vi "CreateLVContextMenu.vi"() -> ()   [LabVIEW 2016]
uses:
  TypeDefs/LV Version Details.ctl
panel:
  out "LV Version Details":T1[](array[typedef])
  in  "Create":bool
  # "The application adds a windows right click context menu for all the versions of LabVIEW\ninstalled on this PC. This makes it handy when you want to open a LabVIEW file in a particular\nversion of LabVIEW instead of the traditional method of File ->Open.\n\nInstructions\n\n1. When you run this application, it lists all the LabVIEW versions installed on this PC.\n2. Clicking on \"Create Context Menus\" button, adds a right click context menu for all the versions.\n3. If you see any erros, check if you are an admin account on this PC or run as admin."
  # "Sample"
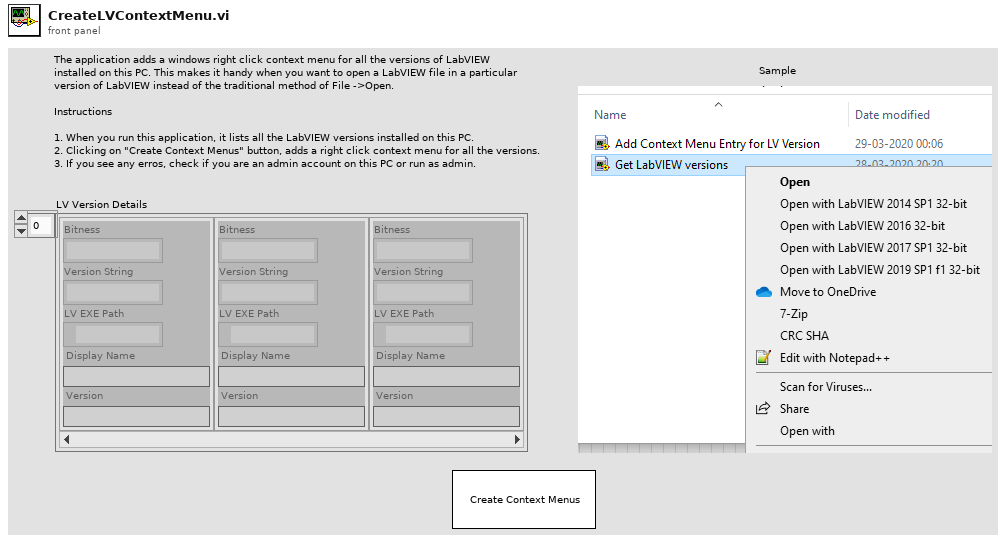
[diagram p1: front panel]
types:
  T1 = typedef "LV Version Details.ctl" = cluster{"Bitness":string, "Version String":string, "LV EXE Path":path, "Display Name":string, "Version":string}
  T2 = enum32{"Invalid", "Standard", "Closed", "Hidden", "Minimized", "Maximized"}
  T3 = enum32{"invalid app kind", "Development System", "Run Time System", "Student Edition", "Embedded LabVIEW", "Evaluation", "Custom"}
  T4 = cluster{"Core":cluster{"Current VI Reference":refnum<vi>, "Close Panel on Exit?":bool}, "Your Boolean data":bool, "Your string data":string, "LV Version Details":T1[]}
  T5 = cluster{"Current VI Reference":refnum<vi>, "Close Panel on Exit?":bool}
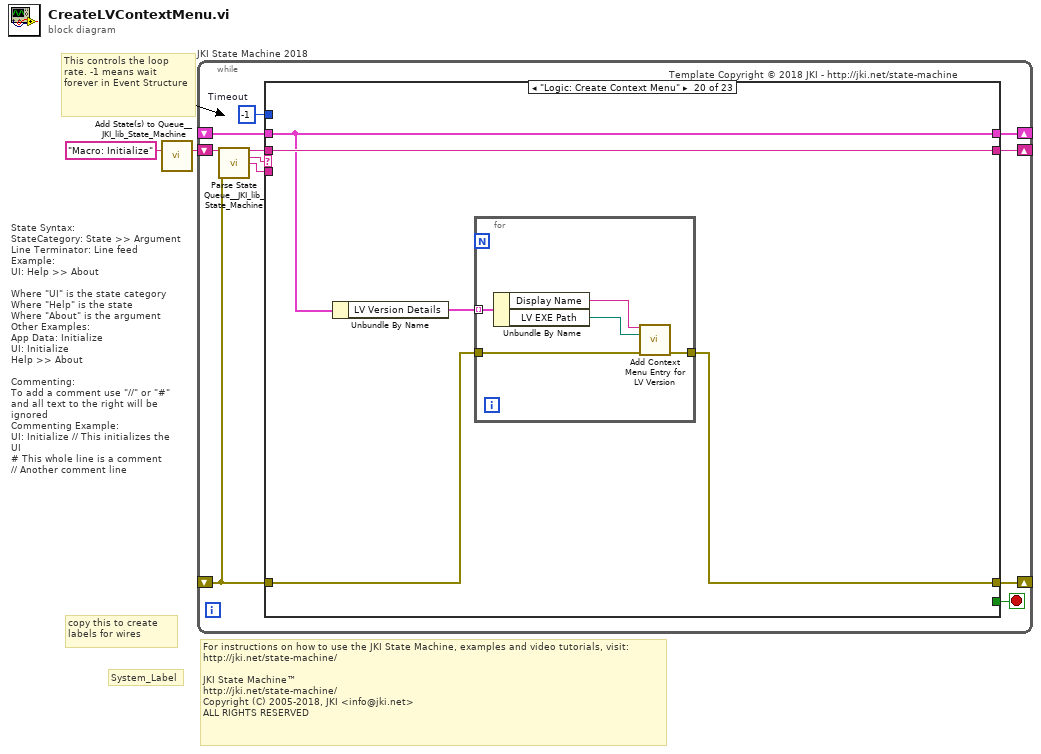
[diagram p0: block diagram]
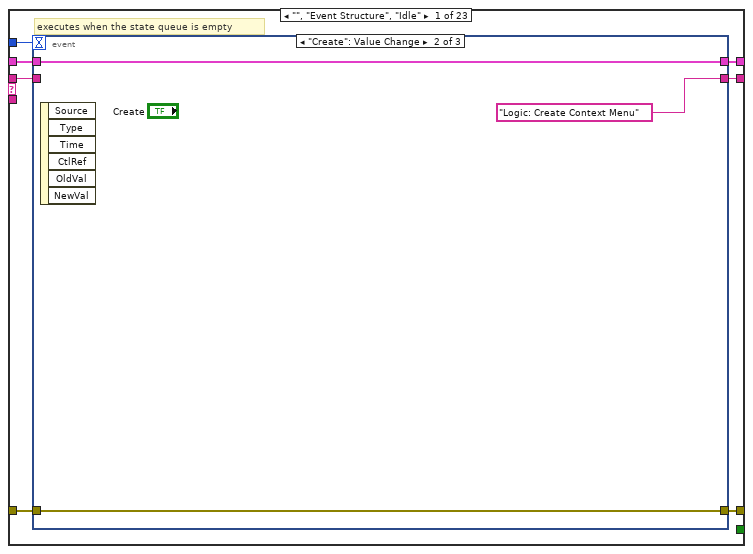
[diagram p2: hidden frame]
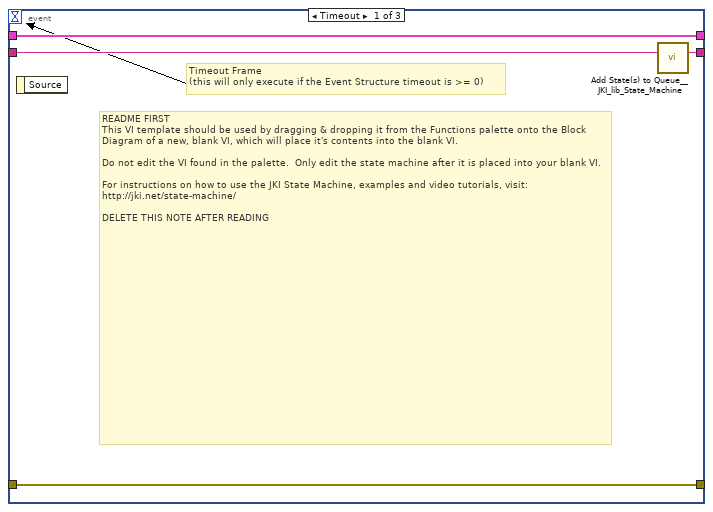
[diagram p3: hidden frame]
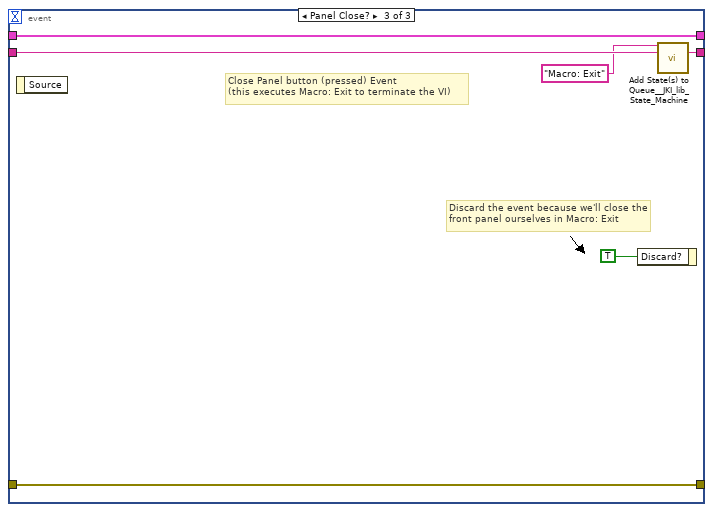
[diagram p4: hidden frame]
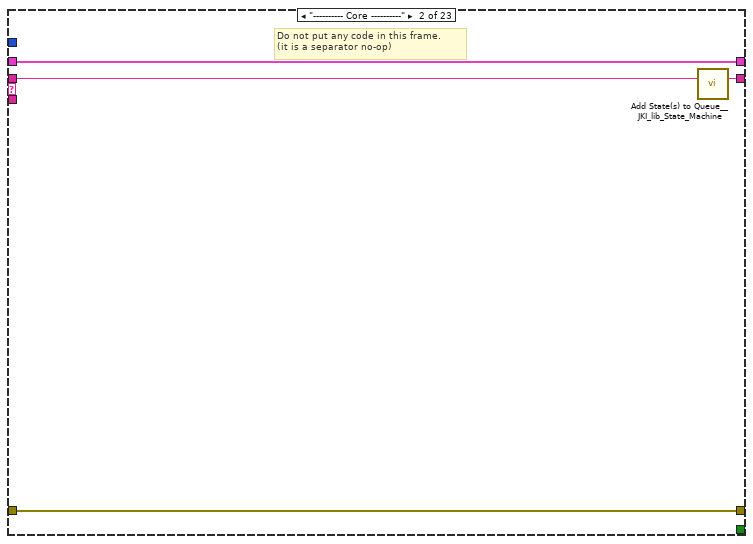
[diagram p5: hidden frame]
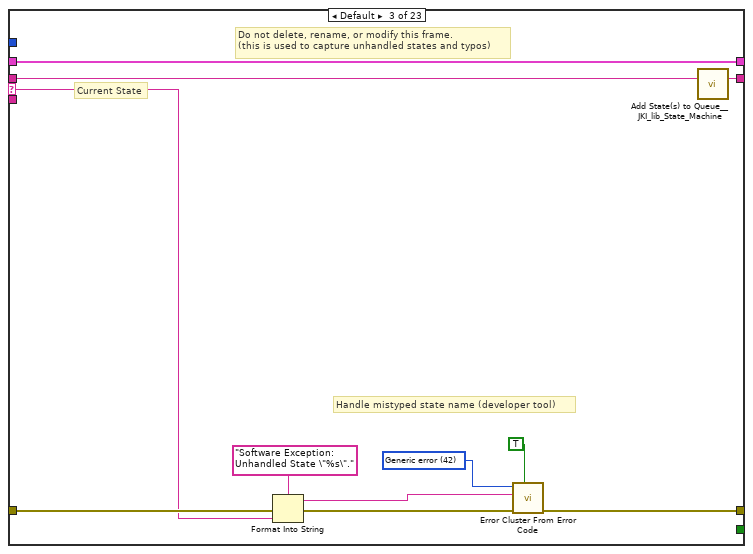
[diagram p6: hidden frame]
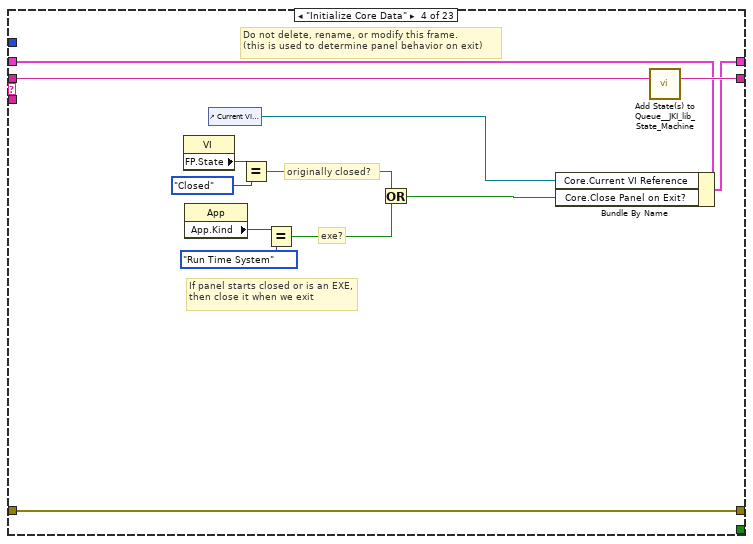
[diagram p7: hidden frame]
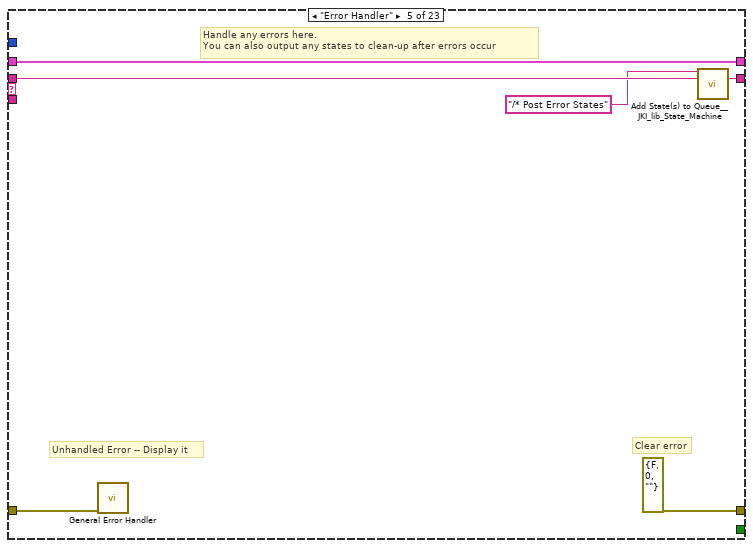
[diagram p8: hidden frame]
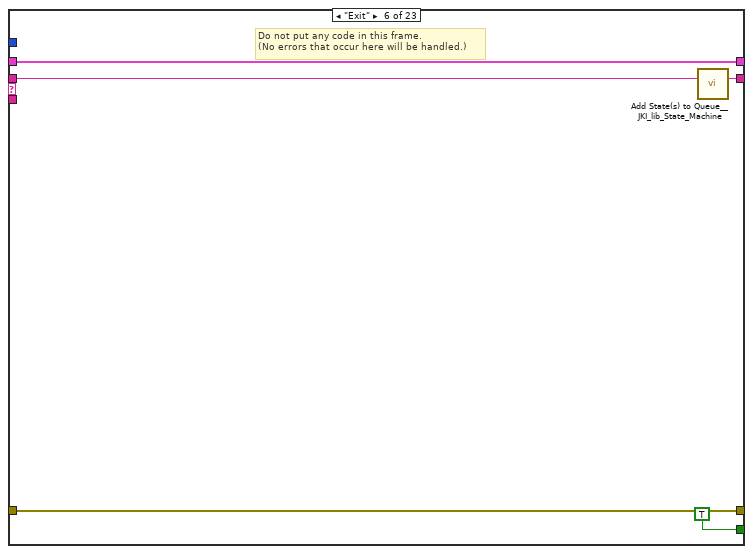
[diagram p9: hidden frame]
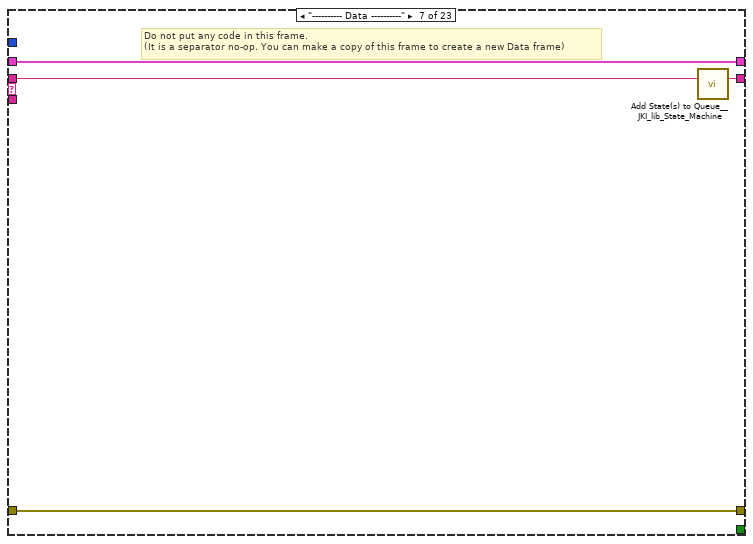
[diagram p10: hidden frame]
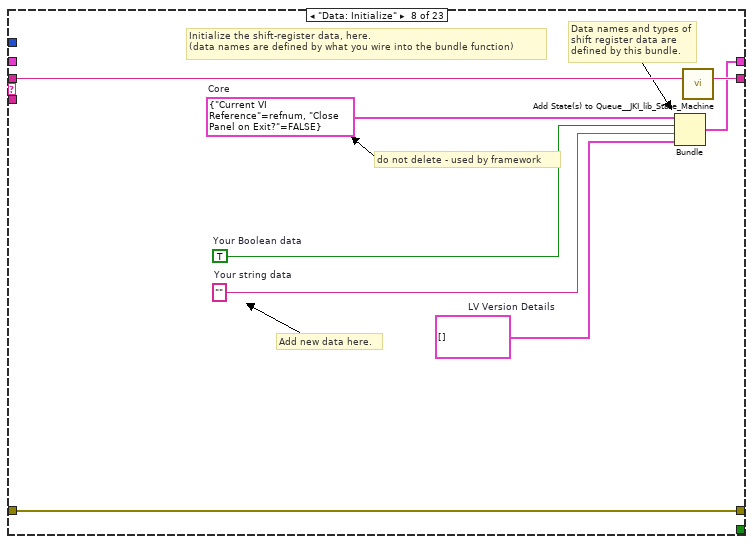
[diagram p11: hidden frame]
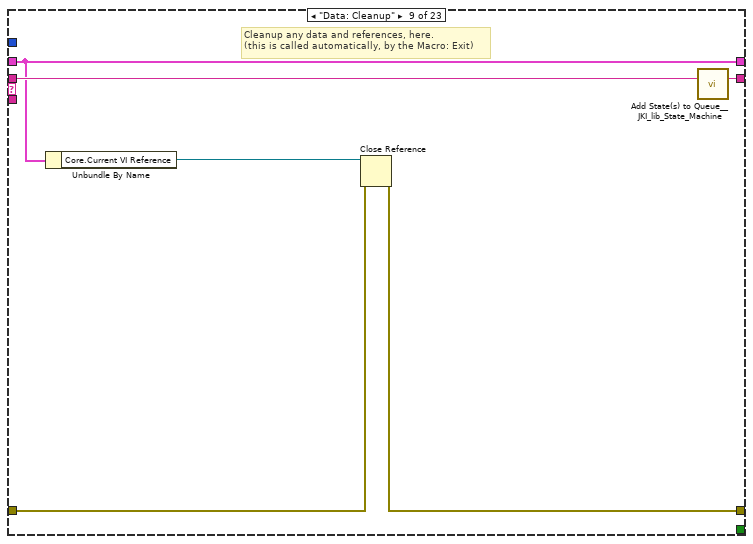
[diagram p12: hidden frame]
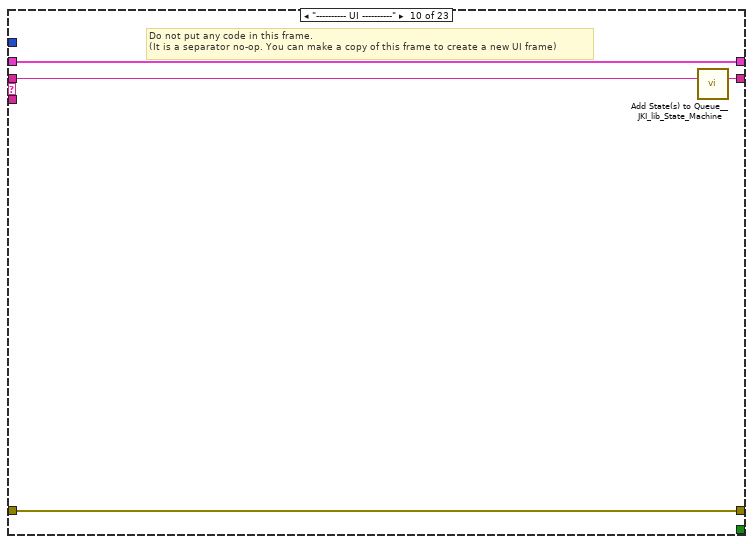
[diagram p13: hidden frame]
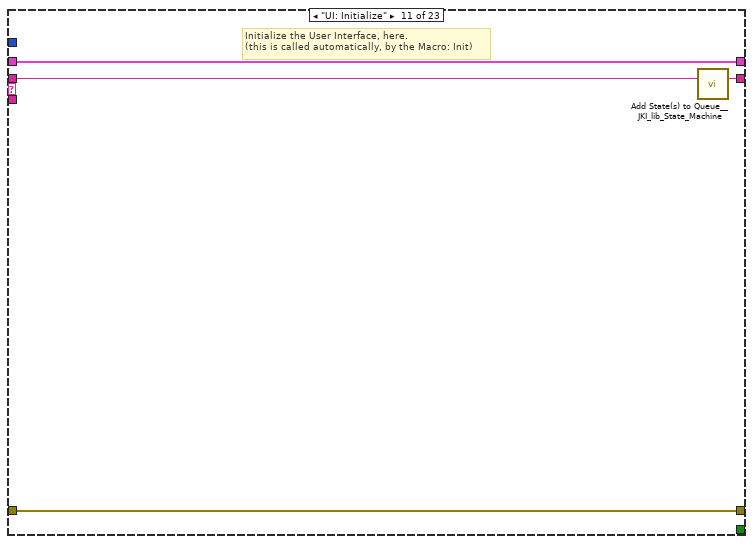
[diagram p14: hidden frame]
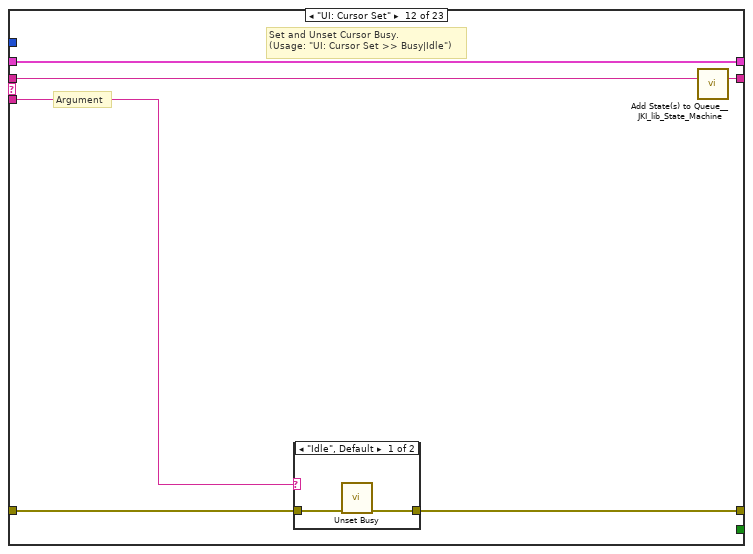
[diagram p15: hidden frame]
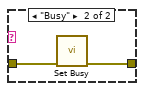
[diagram p16: hidden frame]
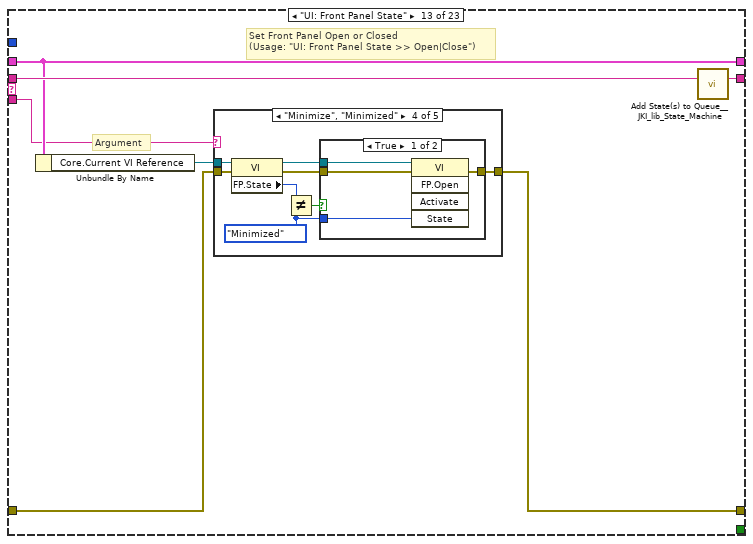
[diagram p17: hidden frame]
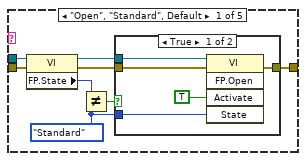
[diagram p18: hidden frame]
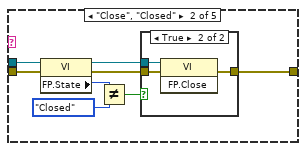
[diagram p20: hidden frame]
diagram:
  # "For instructions on how to use the JKI State Machine, examples and video tutorials, visit:\nhttp://jki.net/state-machine/\n\nJKI State Machine™\nhttp://jki.net/state-machine/\nCopyright (C) 2005-2018, JKI <info@jki.net>\nALL RIGHTS RESERVED"
  # "State Syntax:\nStateCategory: State >> Argument\nLine Terminator: Line feed\nExample:\nUI: Help >> About\n\nWhere \"UI\" is the state category\nWhere \"Help\" is the state\nWhere \"About\" is the argument\nOther Examples:\nApp Data: Initialize\nUI: Initialize\nHelp >> About\n\nCommenting:\nTo add a comment use \"//\" or \"#\" and all text to the right will be ignored\nCommenting Example:\nUI: Initialize // This initializes the UI\n# This whole line is a comment\n// Another comment line"
  # "copy this to create labels for wires"
  # "This controls the loop rate. -1 means wait forever in Event Structure"
  # "System_Label"
  n1 = call <vilib>:"Add State(s) to Queue__JKI_lib_State_Machine.vi"("State(s) in (\"\")"="Macro: Initialize") -> ("States Out"=w2:string)  [unwired: 14 in]
  n2 = while "JKI State Machine 2018" {
    shift-right: [w6] -> _
    shift-left: _ -> [w5]
    shift-right: [w9] -> _
    shift-left: _ -> [w3]
    shift-right: [w8] -> _
    shift-left: w2 -> [w10]
    stop <- w7 stop-if-true
    w4 = -1  # Timeout
    # "Template Copyright © 2018 JKI - http://jki.net/state-machine"
    n3 = call <vilib>:"Parse State Queue__JKI_lib_State_Machine.vi"("State Queue"=w10, "Error In (no error)"=w3) -> ("Remaining States"=w12:string, "Current State"=w13:string, "Arguments"=w11:string)  [unwired: 11 in]
    n4 = case shown="\"Logic: Create Context Menu\"" w13 {
      selector: w13 -> [_ _ w38 _ _ _ _ _ _ _ _ _ _ _ _ _ _ _ _ _ _ _ _]
      tunnel: w12 -> [w20 w37 w42 w61 w67 w72 w76 w84 w90 w94 w98 w104 w115 w183 w188 w193 w203 w205 _ w217 w226 w230 w234]
      tunnel: w11 -> [_ _ _ _ _ _ _ _ _ _ _ w99 w109 _ _ _ _ _ _ _ _ _ _]
      tunnel: w5 -> [w18 w34 w40 w54 w64 w70 w73 _ w85 w91 w96 w102 w111 w182 w185 w190 w200 w206 w209 w216 w223 w227 w231]
      tunnel: [w17 w35 w44 w58 errorcluster {"status"=FALSE, "code"=0, "source"=""} ("error out") w69 w74 w81 w86 w92 w95 w100 w112 w184 w186 w191 w201 w204 w211 w213 w224 w228 w232] -> w9
      tunnel: w3 -> [w16 w35 w43 w58 w63 w69 w74 w81 w87 w92 w95 w101 w113 w184 w186 w191 w201 w204 w212 w215 w224 w228 w232]
      tunnel: [w19 w36 w41 w60 w66 w71 w75 w83 w89 w93 w97 w103 w114 w183 w187 w192 w202 w205 "UI: Display All LabVIEW Versions" w217 w225 w229 w233] -> w8
      tunnel: [_ _ _ _ _ TRUE _ _ _ _ _ _ _ _ _ _ _ _ _ _ _ _ _] -> w7
      tunnel: [w15 w34 w40 w59 w64 w70 w73 w82 w85 w91 w96 w102 w111 w182 w185 w190 w200 w206 w208 w216 w223 w227 w231] -> w6
      tunnel: w4 -> [w14 _ _ _ _ _ _ _ _ _ _ _ _ _ _ _ _ _ _ _ _ _ _]
      frame "", "Event Structure", "Idle" {
        # "executes when the state queue is empty"
        n5 = event shown="[1] \"Create\": Value Change" {
          selector: _ -> [_ _ _]
          dyn-events: _ -> [_ _ _]
          timeout: w14 -> [_ _ _]
          tunnel: w20 -> [w24 _ w33]
          tunnel: [w23 "Logic: Create Context Menu" ("States Out") w32] -> w19
          tunnel: w18 -> [w21 w26 w30]
          tunnel: [w22 w27 w31] -> w17
          tunnel: w16 -> [w22 w27 w31]
          tunnel: [w21 w26 w30] -> w15
          event Timeout {
            # "README FIRST\nThis VI template should be used by dragging & dropping it from the Functions palette onto the Block Diagram of a new, blank VI, which will place it's contents into the blank VI.\n\nDo not edit the VI found in the palette.  Only edit the state machine after it is placed into your blank VI.\n\nFor instructions on how to use the JKI State Machine, examples and video tutorials, visit:\nhttp://jki.net/state-machine/\n\nDELETE THIS NOTE AFTER READING"
            # "Timeout Frame\n(this will only execute if the Event Structure timeout is >= 0)"
            n6 = event-data() -> ()  [unwired: 1 in, 1 out]
            n7 = call <vilib>:"Add State(s) to Queue__JKI_lib_State_Machine.vi"("State(s) in (\"\")"=w24) -> ("States Out"=w23:string)  [unwired: 14 in]
          }
          event "Create": Value Change {
            n8 = event-data() -> ()  [unwired: 1 in, 6 out]
          }
          event Panel Close? {
            # "Discard the event because we'll close the front panel ourselves in Macro: Exit"
            # "Close Panel button (pressed) Event\n(this executes Macro: Exit to terminate the VI)"
            n9 = event-data() -> ()  [unwired: 1 in, 1 out]
            n10 = event-data("Discard?"=TRUE) -> ()  [unwired: 1 in, 1 out]
            n11 = call <vilib>:"Add State(s) to Queue__JKI_lib_State_Machine.vi"("State(s) in Front (\"\")"="Macro: Exit", "State(s) in (\"\")"=w33) -> ("States Out"=w32:string)  [unwired: 13 in]
          }
        }
      }
      frame "---------- Core ----------" {
        # "Do not put any code in this frame.\n(it is a separator no-op)"
        n12 = call <vilib>:"Add State(s) to Queue__JKI_lib_State_Machine.vi"("State(s) in (\"\")"=w37) -> ("States Out"=w36:string)  [unwired: 14 in]
      }
      frame Default {
        w47 = 42 items=["No error", "Argument error", "Memory is full", "Out of zone", "End of file", "File already open", "Generic file I/O error", "File not found", "File permission error", "Disk is full", "Duplicate path", "Too many files open", "System feature not enabled", "Resource file not found", "Cannot add resource", "Resource not found", "Image not found", "Image memory error", "Pen does not exist", "Config type invalid", "Config token not found", "Config parse error", "Config memory error", "Bad external code format", "Bad external code offset", "External code not present", "Null window", "Destroy window error", "Null menu", "Print aborted", "Bad print record", "Print driver error", "Windows error during printing", "Memory error during printing", "Print dialog error", "Generic print error", "Invalid device refnum", "Device not found", "Device parameter error", "Device unit error", "Cannot open device", "Device call aborted", "Generic error", "Cancelled by user", "Object ID too low", "Object ID too high", "Object not in heap", "Unknown heap", "Unknown object (invalid DefProc)", "Unknown object (DefProc not in table)", "Message out of range", "Invalid (null) method", "Unknown message", "Manager call not supported", "Bad address", "Network operation in progress", "Network operation timed out", "Connection is busy", "Network attribute not supported", "Network error", "Address in use", "System out of memory", "Connection aborted", "Connection refused", "Not connected", "Already connected", "Connection closed", "Initialization error (interapplication manager)", "Bad occurrence", "Wait on unbound occurrence handler", "Occurrence queue overflow", "Datalog type conflict", "Unused", "Unrecognized type (interapplication manager)", "Memory corrupt", "Failed to make temporary DLL", "Old CIN version", "Drag socket not found", "Failed to load drop-object", "Failed to register OLE object", "Failed to release OLE object", "Format specifier type mismatch", "Unknown format specifier", "Too few format specifiers", "Too many format specifiers", "Scan failed", "Newer CIN version", "Error converting to variant", "Runtime menu error", "Password tampered", "Variant attribute not found", "Incompatible variant data type", "Event data is not available", "Event Store is not present", "Occurrence is not found", "Event Queue is not created", "Event info is not available", "Refnum passed is NULL", "Error retrieving Class GUID", "Error retrieving CoClass GUID", "Error retrieving TypeLib GUID.", "Bad built application magic bytes.", "Specific driver is different from the specific driver associated with the Logical Name.", "There is no session opened to the class driver.", "Max Error", "MAX - Error with config objects", "MAX - Error loading configuration", "MAX - Group not supported"]
        # "Current State"
        # "Do not delete, rename, or modify this frame.\n(this is used to capture unhandled states and typos)"
        # "Handle mistyped state name (developer tool)"
        n13 = Format Into String(format string="Software Exception: Unhandled State \"%s\"." ("message"), error in=w43, w38) -> (resulting string=w46:string, error out=w45:errorcluster)  [unwired: 1 in]
        n14 = call <vilib>:"Error Cluster From Error Code.vi"("show call chain? (False)"=TRUE, "error in (no error)"=w45, "error message (\"\")"=w46, "error code (0)"=w47) -> ("error out"=w44:errorcluster)  [unwired: 5 in]
        n15 = call <vilib>:"Add State(s) to Queue__JKI_lib_State_Machine.vi"("State(s) in (\"\")"=w42) -> ("States Out"=w41:string)  [unwired: 14 in]
      }
      frame "Initialize Core Data" {
        # "Do not delete, rename, or modify this frame.\n(this is used to determine panel behavior on exit)"
        # "originally closed?"
        # "exe?"
        # "If panel starts closed or is an EXE, then close it when we exit"
        n16 = property class="VI"() -> ("FP.State"=w51:T2)  [unwired: 2 in, 2 out]
        n17 = property class="App"() -> ("App.Kind"=w57:T3)  [unwired: 2 in, 2 out]
        n18 = control-ref of="Current VI Reference"() -> (w52:refnum<vi>)
        n19 = Equal?(x=w51, y=T2."Closed" ("Front Panel Window:State")) -> (x = y?=w49:bool)
        n20 = Equal?(x=w57, y=T3."Run Time System" ("Application:Kind")) -> (x = y?=w55:bool)
        n21 = Or(x=w49, y=w55) -> (x .or. y?=w53:bool)
        n22 = Bundle By Name(cluster=w54, "Core.Current VI Reference"=w52, "Core.Close Panel on Exit?"=w53) -> (w59:T4)
        n23 = call <vilib>:"Add State(s) to Queue__JKI_lib_State_Machine.vi"("State(s) in (\"\")"=w61) -> ("States Out"=w60:string)  [unwired: 14 in]
      }
      frame "Error Handler" {
        # "Unhandled Error -- Display it"
        # "Handle any errors here.\nYou can also output any states to clean-up after errors occur"
        # "Clear error"
        n24 = call <vilib>:"General Error Handler.vi"("error in (no error)"=w63) -> ()  [unwired: 10 in, 5 out]
        n25 = call <vilib>:"Add State(s) to Queue__JKI_lib_State_Machine.vi"("State(s) in Front (\"\")"="/* Post Error States", "State(s) in (\"\")"=w67) -> ("States Out"=w66:string)  [unwired: 13 in]
      }
      frame "Exit" {
        # "Do not put any code in this frame.\n(No errors that occur here will be handled.)"
        n26 = call <vilib>:"Add State(s) to Queue__JKI_lib_State_Machine.vi"("State(s) in (\"\")"=w72) -> ("States Out"=w71:string)  [unwired: 14 in]
      }
      frame "---------- Data ----------" {
        # "Do not put any code in this frame.\n(It is a separator no-op. You can make a copy of this frame to create a new Data frame)"
        n27 = call <vilib>:"Add State(s) to Queue__JKI_lib_State_Machine.vi"("State(s) in (\"\")"=w76) -> ("States Out"=w75:string)  [unwired: 14 in]
      }
      frame "Data: Initialize" {
        w77 = T1[] []  # LV Version Details
        w78 = T5 {"Current VI Reference"=refnum, "Close Panel on Exit?"=FALSE}  # Core
        w80 = TRUE  # Your Boolean data
        w79 = ""  # Your string data
        # "do not delete - used by framework"
        # "Add new data here."
        # "Data names and types of shift register data are defined by this bundle."
        # "Initialize the shift-register data, here.\n(data names are defined by what you wire into the bundle function)"
        n28 = Bundle("Core"=w78, "Your Boolean data"=w80, "Your string data"=w79, "LV Version Details"=w77) -> (w82:T4)  [unwired: 1 in]
        n29 = call <vilib>:"Add State(s) to Queue__JKI_lib_State_Machine.vi"("State(s) in (\"\")"=w84) -> ("States Out"=w83:string)  [unwired: 14 in]
      }
      frame "Data: Cleanup" {
        # "Cleanup any data and references, here.\n(this is called automatically, by the Macro: Exit)"
        n30 = Unbundle By Name(w85) -> ("Core.Current VI Reference"=w88:refnum<vi>)
        n31 = Close Reference(reference=w88, error in (no error)=w87) -> (error out=w86:errorcluster)
        n32 = call <vilib>:"Add State(s) to Queue__JKI_lib_State_Machine.vi"("State(s) in (\"\")"=w90) -> ("States Out"=w89:string)  [unwired: 14 in]
      }
      frame "---------- UI ----------" {
        # "Do not put any code in this frame.\n(It is a separator no-op. You can make a copy of this frame to create a new UI frame)"
        n33 = call <vilib>:"Add State(s) to Queue__JKI_lib_State_Machine.vi"("State(s) in (\"\")"=w94) -> ("States Out"=w93:string)  [unwired: 14 in]
      }
      frame "UI: Initialize" {
        # "Initialize the User Interface, here.\n(this is called automatically, by the Macro: Init)"
        n34 = call <vilib>:"Add State(s) to Queue__JKI_lib_State_Machine.vi"("State(s) in (\"\")"=w98) -> ("States Out"=w97:string)  [unwired: 14 in]
      }
      frame "UI: Cursor Set" {
        # "Argument"
        # "Set and Unset Cursor Busy.\n(Usage: \"UI: Cursor Set >> Busy|Idle\")"
        n35 = case shown="\"Idle\", Default" w99 {
          tunnel: w101 -> [w106 w108]
          tunnel: [w105 w107] -> w100
          frame "Idle", Default {
            n36 = call <vilib>:"Unset Busy.vi"("error in (no error)"=w106) -> ("error out"=w105:errorcluster)  [unwired: 10 in]
          }
          frame "Busy" {
            n37 = call <vilib>:"Set Busy.vi"("error in (no error)"=w108) -> ("error out"=w107:errorcluster)  [unwired: 9 in, 1 out]
          }
        }
        n38 = call <vilib>:"Add State(s) to Queue__JKI_lib_State_Machine.vi"("State(s) in (\"\")"=w104) -> ("States Out"=w103:string)  [unwired: 14 in]
      }
      frame "UI: Front Panel State" {
        # "Argument"
        # "Set Front Panel Open or Closed\n(Usage: \"UI: Front Panel State >> Open|Close\")"
        n39 = Unbundle By Name(w111) -> ("Core.Current VI Reference"=w110:refnum<vi>)
        n40 = case shown="\"Minimize\", \"Minimized\"" w109 {
          tunnel: w113 -> [w121 w136 w147 w160 w173]
          tunnel: [w123 w137 w149 w162 w175] -> w112
          tunnel: w110 -> [w122 w134 w148 w161 w174]
          frame "Open", "Standard", Default {
            w116 = T2."Standard" ("State")
            n41 = property class="VI"(reference=w122, error in=w121) -> (reference out=w119:refnum<vi>, error out=w120:errorcluster, "FP.State"=w118:T2)
            n42 = Not Equal?(x=w118, y=w116) -> (x != y?=w117:bool)
            n43 = case shown="True" w117 {
              tunnel: [w127 w129] -> w123
              tunnel: w120 -> [w126 w129]
              tunnel: w119 -> [w125 _]
              tunnel: w116 -> [w124 _]
              frame True {
                n44 = invoke class="VI" method="FP.Open"(reference=w125, error in=w126, "Activate"=TRUE, "State"=w124) -> (error out=w127:errorcluster)  [unwired: 1 in, 4 out]
              }
              frame False {
              }
            }
          }
          frame "Close", "Closed" {
            n45 = property class="VI"(reference=w134, error in=w136) -> (reference out=w133:refnum<vi>, error out=w135:errorcluster, "FP.State"=w131:T2)
            n46 = Not Equal?(x=w131, y=T2."Closed" ("Front Panel Window:State")) -> (x != y?=w130:bool)
            n47 = case shown="True" w130 {
              tunnel: [w138 w141] -> w137
              tunnel: w135 -> [w138 w140]
              tunnel: w133 -> [_ w139]
              frame False {
              }
              frame True {
                n48 = invoke class="VI" method="FP.Close"(reference=w139, error in=w140) -> (error out=w141:errorcluster)  [unwired: 1 in, 2 out]
              }
            }
          }
          frame "Hidden", "Hide" {
            w142 = T2."Hidden" ("State")
            n49 = property class="VI"(reference=w148, error in=w147) -> (reference out=w145:refnum<vi>, error out=w146:errorcluster, "FP.State"=w144:T2)
            n50 = Not Equal?(x=w144, y=w142) -> (x != y?=w143:bool)
            n51 = case shown="True" w143 {
              tunnel: [w153 w154] -> w149
              tunnel: w146 -> [w152 w154]
              tunnel: w145 -> [w151 _]
              tunnel: w142 -> [w150 _]
              frame True {
                n52 = invoke class="VI" method="FP.Open"(reference=w151, error in=w152, "State"=w150) -> (error out=w153:errorcluster)  [unwired: 2 in, 4 out]
              }
              frame False {
              }
            }
          }
          frame "Minimize", "Minimized" {
            w155 = T2."Minimized" ("State")
            n53 = property class="VI"(reference=w161, error in=w160) -> (reference out=w158:refnum<vi>, error out=w159:errorcluster, "FP.State"=w157:T2)
            n54 = Not Equal?(x=w157, y=w155) -> (x != y?=w156:bool)
            n55 = case shown="True" w156 {
              tunnel: [w166 w167] -> w162
              tunnel: w159 -> [w165 w167]
              tunnel: w158 -> [w164 _]
              tunnel: w155 -> [w163 _]
              frame True {
                n56 = invoke class="VI" method="FP.Open"(reference=w164, error in=w165, "State"=w163) -> (error out=w166:errorcluster)  [unwired: 2 in, 4 out]
              }
              frame False {
              }
            }
          }
          frame "Maximize", "Maximized" {
            w168 = T2."Maximized" ("State")
            n57 = property class="VI"(reference=w174, error in=w173) -> (reference out=w171:refnum<vi>, error out=w172:errorcluster, "FP.State"=w170:T2)
            n58 = Not Equal?(x=w170, y=w168) -> (x != y?=w169:bool)
            n59 = case shown="True" w169 {
              tunnel: [w179 w180] -> w175
              tunnel: w172 -> [w178 w180]
              tunnel: w171 -> [w177 _]
              tunnel: w168 -> [w176 _]
              frame True {
                n60 = invoke class="VI" method="FP.Open"(reference=w177, error in=w178, "State"=w176) -> (error out=w179:errorcluster)  [unwired: 2 in, 4 out]
              }
              frame False {
              }
            }
          }
        }
        n61 = call <vilib>:"Add State(s) to Queue__JKI_lib_State_Machine.vi"("State(s) in (\"\")"=w115) -> ("States Out"=w114:string)  [unwired: 14 in]
      }
      frame "UI: Display All LabVIEW Versions" {
        n62 = Unbundle By Name(w182) -> ("LV Version Details"=→"LV Version Details":T1[])
      }
      frame "---------- Macro ----------" {
        # "Do not put any code in this frame.\n(It is a separator no-op. You can make a copy of this frame to create a new Macro frame)"
        n63 = call <vilib>:"Add State(s) to Queue__JKI_lib_State_Machine.vi"("State(s) in (\"\")"=w188) -> ("States Out"=w187:string)  [unwired: 14 in]
      }
      frame "Macro: Initialize" {
        w189 = "Data: Initialize\nInitialize Core Data\nUI: Initialize\nUI: Front Panel State >> Open\nLogic: Get All LabVIEW Versions"  # Data: Initialize Initialize Core Data UI: Initialize UI: Front Panel State >> Open Logic: Get All LabVIEW Versions
        # "Initialization Macro\n(This is called once, when the VI starts)"
        n64 = call <vilib>:"Add State(s) to Queue__JKI_lib_State_Machine.vi"("State(s) in Front (\"\")"=w189, "State(s) in (\"\")"=w193) -> ("States Out"=w192:string)  [unwired: 13 in]
      }
      frame "Macro: Exit" {
        # "Exit Macro\n(This is called once, when the VI exits)"
        n65 = Unbundle By Name(w200) -> ("Core.Close Panel on Exit?"=w199:bool)
        n66 = Select(t="UI: Front Panel State >> Close", s=w199, f="") -> (s? t:f=w196:string)
        n67 = call <vilib>:"Add State(s) to Queue__JKI_lib_State_Machine.vi"("State(s) in (\"\")"=w196, "State(s) at Back (\"\")"="Data: Cleanup\nExit") -> ("States Out"=w194:string)  [unwired: 13 in]
        n68 = call <vilib>:"Add State(s) to Queue__JKI_lib_State_Machine.vi"("State(s) in Front (\"\")"=w194, "State(s) in (\"\")"=w203) -> ("States Out"=w202:string)  [unwired: 13 in]
      }
      frame "-----------Logic-----------------" {
      }
      frame "Logic: Get All LabVIEW Versions" {
        n69 = call "Get LabVIEW versions.vi"("error in (no error)"=w212) -> ("error out"=w211:errorcluster, "LV Version Details"=w207:T1[])  [unwired: 9 in]
        n70 = Bundle By Name(cluster=w209, "LV Version Details"=w207) -> (w208:T4)
      }
      frame "Logic: Create Context Menu" {
        n71 = Unbundle By Name(w216) -> ("LV Version Details"=w214:T1[])
        n72 = for {
          tunnel: w215 -> [w222]
          tunnel: [w221] -> w213
          tunnel: w214 -> [w220] mode=indexing
          n73 = Unbundle By Name(w220) -> ("Display Name"=w219:string, "LV EXE Path"=w218:path)
          n74 = call "Add Context Menu Entry for LV Version.vi"("LabVIEW Version String"=w219, "LabVIEW EXE Path"=w218, "error in (no error)"=w222) -> ("error out"=w221:errorcluster)  [unwired: 12 in]
        }
      }
      frame "---------- New Category ----------" {
        # "Template Separator\n(You can make a copy of, or modify, this frame)"
        n75 = call <vilib>:"Add State(s) to Queue__JKI_lib_State_Machine.vi"("State(s) in (\"\")"=w226) -> ("States Out"=w225:string)  [unwired: 14 in]
      }
      frame "New Category: 1" {
        # "Your code here.\n(You can make a copy of, or modify, this frame)"
        n76 = call <vilib>:"Add State(s) to Queue__JKI_lib_State_Machine.vi"("State(s) in (\"\")"=w230) -> ("States Out"=w229:string)  [unwired: 14 in]
      }
      frame "New Category: 2" {
        # "Your code here.\n(You can make a copy of, or modify, this frame)"
        n77 = call <vilib>:"Add State(s) to Queue__JKI_lib_State_Machine.vi"("State(s) in (\"\")"=w234) -> ("States Out"=w233:string)  [unwired: 14 in]
      }
    }
  }
